vi "Finish.vi"   [LabVIEW 2016]
doc: "This VI is called just before exiting. It is expected to close I/O refnum, save collected data, etc."
uses:
  <vilib>/Rock Robotics/WPI/Utilities/WPI_GetSetVariantRefNum.vi
types:
  T1 = typedef "WPI_MotorControlDeviceRef.ctl" = cluster{"DeviceStatus":errorcluster, "Type":T2, "PWM":cluster{"PWM Channel":T3, "DeadBand":T4}, "CAN":cluster{"Device Number":u8, "SetOutput VI Ref":variant, "GetOutput VI Ref":variant, "Enable VI Ref":variant, "Disable VI Ref":variant, "Data":variant}, "Invert":bool}
  T2 = typedef "WPI_MotorControlType.ctl" = enum16{"PWM", "CAN"}
  T3 = typedef "FPGA_DIOPWMChannel.ctl" = enum8{"PWM 0", "PWM 1", "PWM 2", "PWM 3", "PWM 4", "PWM 5", "PWM 6", "PWM 7", "PWM 8", "PWM 9", "PWM MXP 0", "PWM MXP 1", "PWM MXP 2", "PWM MXP 3", "PWM MXP 4", "PWM MXP 5", "PWM MXP 6", "PWM MXP 7", "PWM MXP 8", "PWM MXP 9", "Invalid"}
  T4 = typedef "WPI_PWMDeadband.ctl" = cluster{"Name":string, "maxPositivePwm":i32, "minPositivePwm":i32, "centerPwm":i32, "maxNegativePwm":i32, "minNegativePwm":i32, "angularRange":u16}
  T5 = typedef "WPI_SolenoidDevRef.ctl" = cluster{"DevStatus":errorcluster, "Pneumatics Control Module":u8, "Forward Solenoid Channel":T6, "Reverse Solenoid Channel":T6}
  T6 = typedef "WPI_SolenoidChannel.ctl" = enum8{"Solenoid 0", "Solenoid 1", "Solenoid 2", "Solenoid 3", "Solenoid 4", "Solenoid 5", "Solenoid 6", "Solenoid 7", "Invalid"}
  T7 = typedef "WPI_RelayDevRef.ctl" = cluster{"DevStatus":errorcluster, "Relay Channel":T8, "Relay Direction":T9}
  T8 = typedef "FPGA_DIORelayChannel.ctl" = enum8{"Relay 0", "Relay 1", "Relay 2", "Relay 3", "Invalid"}
  T9 = typedef "WPI_RelayDirection.ctl" = enum16{"Both directions", "Forward only", "Reverse only"}
  T10 = typedef "WPI_JoystickDevRef.ctl" = cluster{"Device":T11}
  T11 = typedef "WPI_JoystickDeviceEnum.ctl" = enum16{"USB 0", "USB 1", "USB 2", "USB 3", "USB 4", "USB 5"}
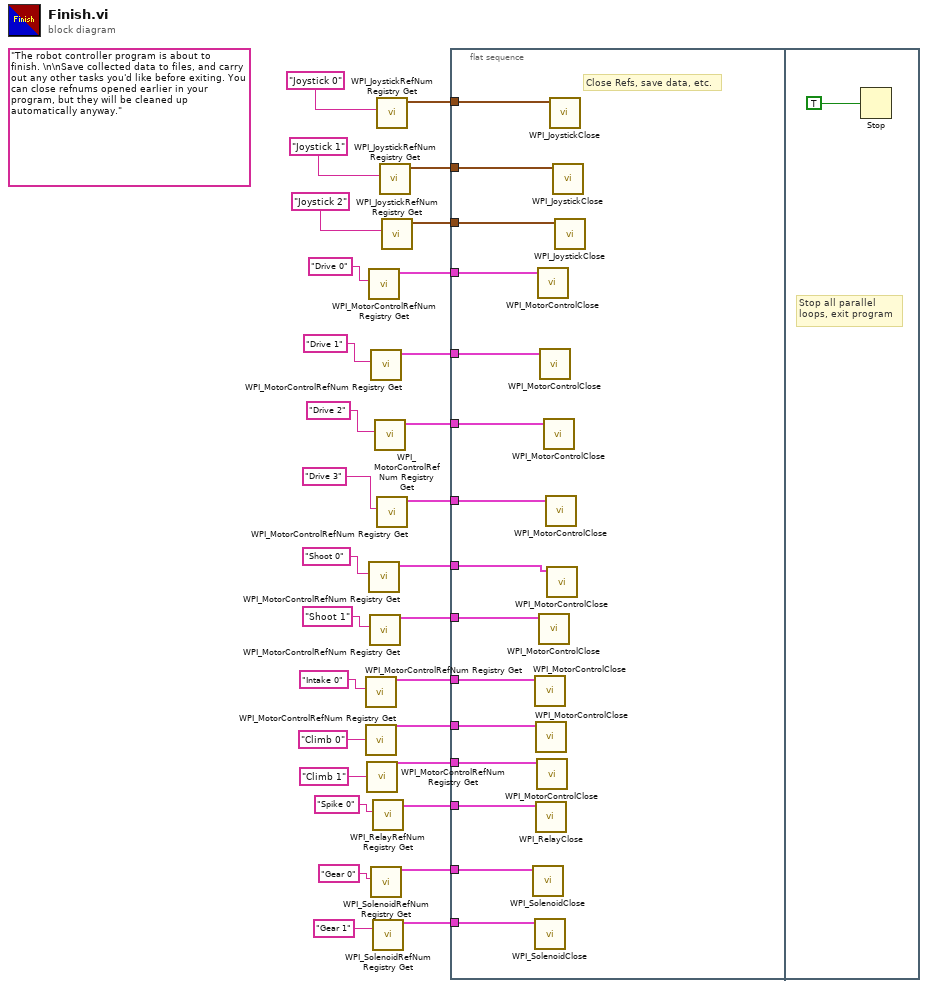
[diagram p0: block diagram]
diagram:
  (unwired) "The robot controller program is about to finish. \n\nSave collected data to files, and carry out any other tasks you'd like before exiting. You can close refnums opened earlier in your program, but they will be cleaned up automatically anyway."
  n1 = call <vilib>:"WPI_MotorControlRefNum Registry Get.vi"("refnum name"="Intake 0") -> ("MotorControlDevRef"=w12:T1)  [unwired: 9 in, 1 out]
  n2 = call <vilib>:"WPI_MotorControlRefNum Registry Get.vi"("refnum name"="Climb 0") -> ("MotorControlDevRef"=w4:T1)  [unwired: 9 in, 1 out]
  n3 = call <vilib>:"WPI_MotorControlRefNum Registry Get.vi"("refnum name"="Climb 1") -> ("MotorControlDevRef"=w1:T1)  [unwired: 9 in, 1 out]
  n4 = call <vilib>:"WPI_MotorControlRefNum Registry Get.vi"("refnum name"="Drive 0") -> ("MotorControlDevRef"=w19:T1)  [unwired: 9 in, 1 out]
  n5 = call <vilib>:"WPI_MotorControlRefNum Registry Get.vi"("refnum name"="Shoot 0") -> ("MotorControlDevRef"=w15:T1)  [unwired: 9 in, 1 out]
  n6 = call <vilib>:"WPI_MotorControlRefNum Registry Get.vi"("refnum name"="Shoot 1") -> ("MotorControlDevRef"=w14:T1)  [unwired: 9 in, 1 out]
  n7 = call <vilib>:"WPI_MotorControlRefNum Registry Get.vi"("refnum name"="Drive 1") -> ("MotorControlDevRef"=w21:T1)  [unwired: 9 in, 1 out]
  n8 = call <vilib>:"WPI_SolenoidRefNum Registry Get.vi"("refnum name"="Gear 0") -> ("SolenoidDevRef"=w7:T5)  [unwired: 9 in, 1 out]
  n9 = call <vilib>:"WPI_RelayRefNum Registry Get.vi"("refnum name"="Spike 0") -> ("RelayDevRef"=w9:T7)  [unwired: 9 in, 1 out]
  n10 = call <vilib>:"WPI_SolenoidRefNum Registry Get.vi"("refnum name"="Gear 1") -> ("SolenoidDevRef"=w6:T5)  [unwired: 9 in, 1 out]
  n11 = call <vilib>:"WPI_MotorControlRefNum Registry Get.vi"("refnum name"="Drive 2") -> ("MotorControlDevRef"=w22:T1)  [unwired: 9 in, 1 out]
  n12 = call <vilib>:"WPI_JoystickRefNum Registry Get.vi"("refnum name"="Joystick 0") -> ("JoystickDevRef"=w29:T10)  [unwired: 1 in, 9 out]
  n13 = call <vilib>:"WPI_MotorControlRefNum Registry Get.vi"("refnum name"="Drive 3") -> ("MotorControlDevRef"=w23:T1)  [unwired: 9 in, 1 out]
  n14 = call <vilib>:"WPI_JoystickRefNum Registry Get.vi"("refnum name"="Joystick 1") -> ("JoystickDevRef"=w28:T10)  [unwired: 1 in, 9 out]
  n15 = call <vilib>:"WPI_JoystickRefNum Registry Get.vi"("refnum name"="Joystick 2") -> ("JoystickDevRef"=w25:T10)  [unwired: 1 in, 9 out]
  n16 = flat-sequence {
    tunnel: w29 -> [w45]
    tunnel: w28 -> [w44]
    tunnel: w25 -> [w43]
    tunnel: w23 -> [w42]
    tunnel: w22 -> [w41]
    tunnel: w21 -> [w40]
    tunnel: w19 -> [w39]
    tunnel: w15 -> [w38]
    tunnel: w14 -> [w37]
    tunnel: w12 -> [w36]
    tunnel: w9 -> [w35]
    tunnel: w7 -> [w34]
    tunnel: w6 -> [w33]
    tunnel: w4 -> [w32]
    tunnel: w1 -> [w31]
    frame #0 {
      # "Close Refs, save data, etc."
      n17 = call <vilib>:"WPI_SolenoidClose.vi"("SolenoidDevRef"=w34) -> ()  [unwired: 10 in, 1 out]
      n18 = call <vilib>:"WPI_MotorControlClose.vi"("MotorControlDevRef"=w36) -> ()  [unwired: 10 in, 1 out]
      n19 = call <vilib>:"WPI_SolenoidClose.vi"("SolenoidDevRef"=w33) -> ()  [unwired: 10 in, 1 out]
      n20 = call <vilib>:"WPI_MotorControlClose.vi"("MotorControlDevRef"=w32) -> ()  [unwired: 10 in, 1 out]
      n21 = call <vilib>:"WPI_RelayClose.vi"("RelayDevRef"=w35) -> ()  [unwired: 10 in, 1 out]
      n22 = call <vilib>:"WPI_MotorControlClose.vi"("MotorControlDevRef"=w31) -> ()  [unwired: 10 in, 1 out]
      n23 = call <vilib>:"WPI_MotorControlClose.vi"("MotorControlDevRef"=w39) -> ()  [unwired: 10 in, 1 out]
      n24 = call <vilib>:"WPI_MotorControlClose.vi"("MotorControlDevRef"=w37) -> ()  [unwired: 10 in, 1 out]
      n25 = call <vilib>:"WPI_MotorControlClose.vi"("MotorControlDevRef"=w40) -> ()  [unwired: 10 in, 1 out]
      n26 = call <vilib>:"WPI_MotorControlClose.vi"("MotorControlDevRef"=w41) -> ()  [unwired: 10 in, 1 out]
      n27 = call <vilib>:"WPI_MotorControlClose.vi"("MotorControlDevRef"=w42) -> ()  [unwired: 10 in, 1 out]
      n28 = call <vilib>:"WPI_MotorControlClose.vi"("MotorControlDevRef"=w38) -> ()  [unwired: 10 in, 1 out]
      n29 = call <vilib>:"WPI_JoystickClose.vi"("JoystickDevRef"=w45) -> ()  [unwired: 11 out]
      n30 = call <vilib>:"WPI_JoystickClose.vi"("JoystickDevRef"=w44) -> ()  [unwired: 11 out]
      n31 = call <vilib>:"WPI_JoystickClose.vi"("JoystickDevRef"=w43) -> ()  [unwired: 11 out]
    }
    frame #1 {
      # "Stop all parallel\nloops, exit program"
      n32 = Stop(stop? (T)=TRUE ("Quit")) -> ()
    }
  }
